vi "WriteUAsub.vi"(0 "OPC UA client refnum in":T1, 9 "error in (no error)":errorcluster, 11 "SetpointID":T2, 12 "TemperatureID":T2, 13 "Setpoint[C]":dbl, 14 "Temperature[C]":dbl) -> (4 "OPC UA client refnum out":T1, 10 "error out":errorcluster)   [LabVIEW 2019]
uses:
  <vilib>/OPCUA/controls/OPC UA Client Refnum.ctl
  <vilib>/OPCUA/controls/NodeId.ctl
  <vilib>/OPCUA/controls/Write Status.ctl
  <vilib>/OPCUA/client/Multiple Write Double.vi
  <vilib>/OPCUA/NI OPC UA Client.lvlib
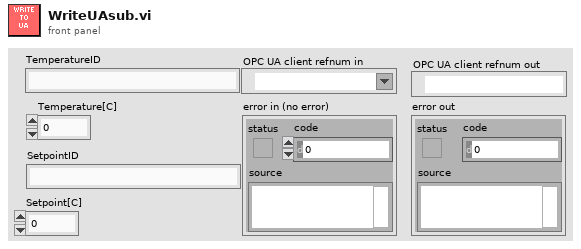
[diagram p1: front panel]
types:
  T1 = typedef "OPC UA Client Refnum.ctl" = refnum<k21>
  T2 = typedef "NodeId.ctl" = string
  T3 = typedef "Write Status.ctl" = u32
  T4 = cluster{"node ID":T2, "value":dbl, "timestamp (current time)":timestamp, "node status":T3}
  T5 = cluster{"node ID":T2, "value":dbl, "timestamp (current time)":timestamp, "node status":T3}[]
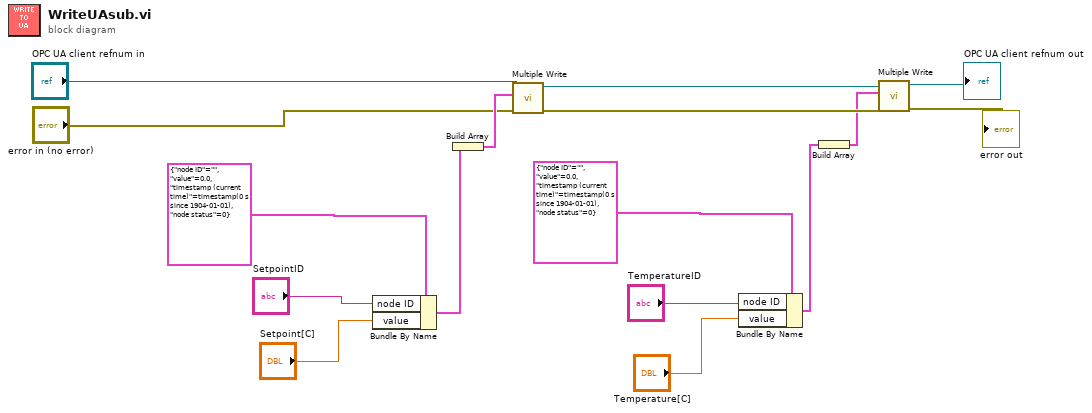
[diagram p0: block diagram]
diagram:
  n1 = Bundle By Name(cluster=T4 {"node ID"="", "value"=0.0, "timestamp (current time)"=timestamp(0 s since 1904-01-01), "node status"=0} ("input cluster"), "node ID"="SetpointID", "value"="Setpoint[C]") -> (w16:T4)
  n2 = Build Array(w16) -> (w15:T5)
  n3 = call-poly <vilib>:"Multiple Write.vi"("error in (no error)"="error in (no error)", "requests"=w15, "OPC UA client refnum in"="OPC UA client refnum in") -> ("error out"=w9:errorcluster, "OPC UA client refnum out"=w10:T1)  [unwired: 5 in, 2 out]
  n4 = Bundle By Name(cluster=T4 {"node ID"="", "value"=0.0, "timestamp (current time)"=timestamp(0 s since 1904-01-01), "node status"=0} ("input cluster"), "node ID"="TemperatureID", "value"="Temperature[C]") -> (w8:T4)
  n5 = Build Array(w8) -> (w7:T5)
  n6 = call-poly <vilib>:"Multiple Write.vi"("error in (no error)"=w9, "requests"=w7, "OPC UA client refnum in"=w10) -> ("error out"=→"error out":errorcluster, "OPC UA client refnum out"=→"OPC UA client refnum out":T1)  [unwired: 5 in, 2 out]
